vi "Data File Names.vi"(8 "error in (no error)":errorcluster, 11 "Data Directory":path=path "C:/Users/plane/Desktop/LabVIEW/Data") -> (0 "error out":errorcluster, 1 "Reduced Data File":path, 2 "Log File":path, 3 "Raw Data File":path)   [LabVIEW 2013, in "Breakdown Acoustics Controls.lvlib"]
uses:
  Breakdown Acoustics Controls.lvlib
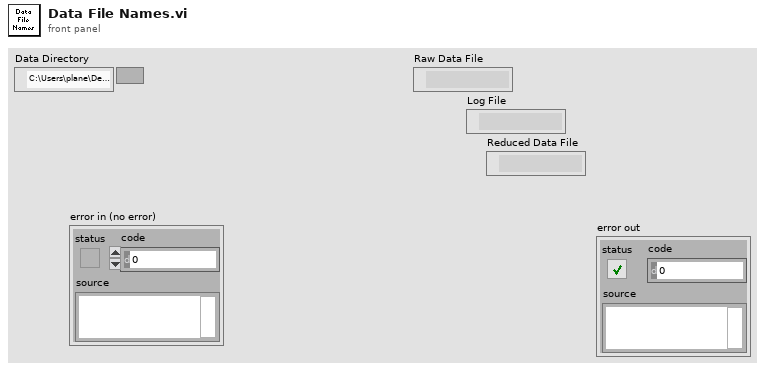
[diagram p1: front panel]
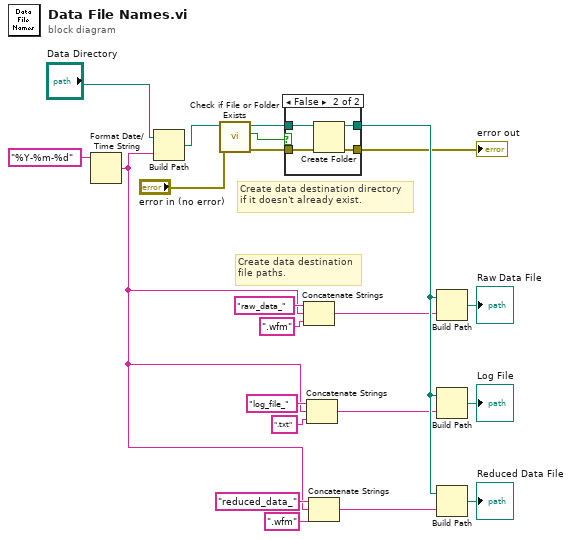
[diagram p0: block diagram]
diagram:
  # "Create data destination\nfile paths."
  # "Create data destination directory\nif it doesn't already exist."
  n1 = Format Date/Time String(time format string (%c)="%Y-%m-%d") -> (date/time string=w9:string)  [unwired: 2 in]
  n2 = Build Path(base path="Data Directory", name or relative path=w9) -> (appended path=w21:path)
  n3 = call <vilib>:"Check if File or Folder Exists.vi"("error in (no error)"="error in (no error)", "path"=w21) -> ("error out"=w18:errorcluster, "file or folder exists?"=w19:bool, "dup path"=w20:path)  [unwired: 7 in]
  n4 = case shown="False" w19 {
    tunnel: w20 -> [w24 w28]
    tunnel: [w24 w27] -> w15
    tunnel: w18 -> [w23 w26]
    tunnel: [w23 w25] -> w1
    frame True {
    }
    frame False {
      n5 = Create Folder(path (use dialog)=w28, error in=w26) -> (created path=w27:path, error out=w25:errorcluster)  [unwired: 1 in, 1 out]
    }
  }
  "error out" <- w1
  n6 = Concatenate Strings("raw_data_" ("string"), w9, ".wfm" ("string")) -> (w7:string)
  n7 = Concatenate Strings("log_file_" ("string"), w9, ".txt" ("string")) -> (w6:string)
  n8 = Concatenate Strings("reduced_data_" ("string"), w9, ".wfm" ("string")) -> (w5:string)
  n9 = Build Path(base path=w15, name or relative path=w7) -> (appended path=→"Raw Data File":path)
  n10 = Build Path(base path=w15, name or relative path=w6) -> (appended path=→"Log File":path)
  n11 = Build Path(base path=w15, name or relative path=w5) -> (appended path=→"Reduced Data File":path)
